vi "3.labtask4 (1).vi"() -> ()   [LabVIEW 2022 SP3]
uses:
  <vilib>/Utility/file.llb/Write Delimited Spreadsheet (DBL).vi
panel:
  out "Array":dbl[](array[numeric])
  in  "file path (dialog if empty)":path
  out "Waveform Chart":dynamicdata(graph)
  out "Total execution time (s)":u32
  out "Sampling period (ms)":dbl
  out "Total number of samples":dbl
  in  "Sampling rate (Hz)":dbl
  in  "Total duration (s)":dbl
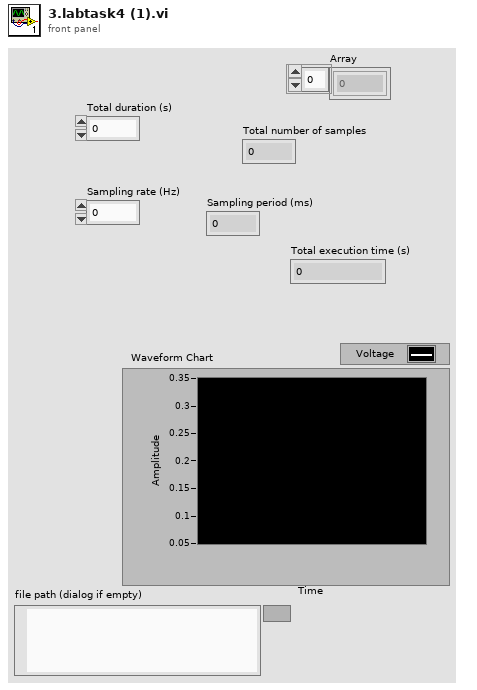
[diagram p1: front panel]
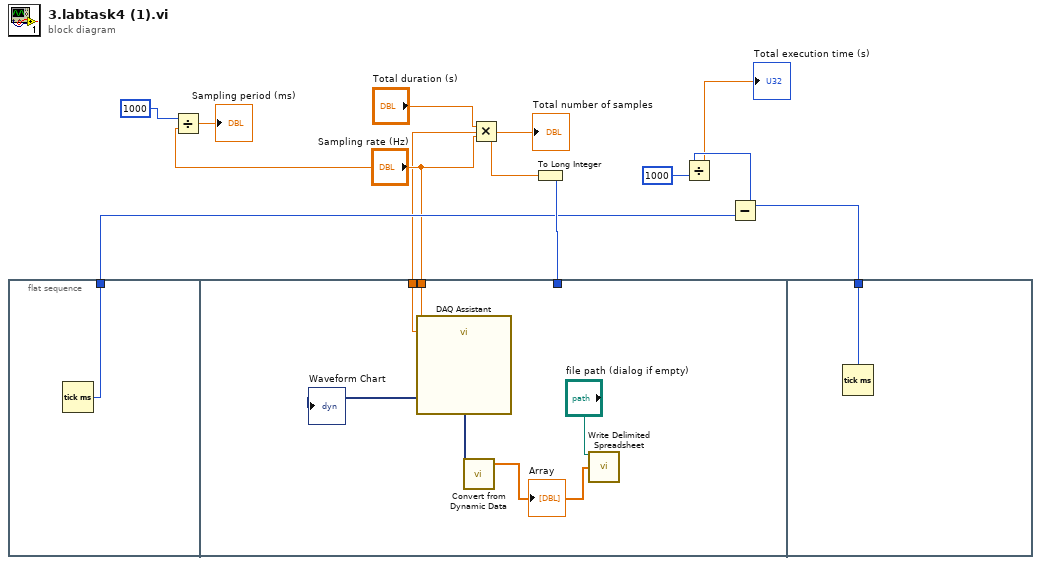
[diagram p0: block diagram]
diagram:
  n1 = flat-sequence {
    tunnel: [w12] -> w4
    tunnel: w9 -> [_]
    tunnel: "Sampling rate (Hz)" -> [w17]
    tunnel: w1 -> [w16]
    tunnel: [w18] -> w5
    frame #0 {
      n2 = Tick Count (ms)() -> (millisecond timer value=w12:u32)
    }
    frame #1 {
      n3 = call "DAQ Assistant"("rate"=w17, "number of samples"=w16) -> ("data"=w13:dynamicdata)  [unwired: 15 in, 2 out]
      "Waveform Chart" <- w13
      n4 = call "Convert from Dynamic Data"("Dynamic Data Type"=w13) -> ("Array"=w14:dbl[])  [unwired: 3 in]
      "Array" <- w14
      n5 = call-poly <vilib>:"Write Delimited Spreadsheet.vi"("file path (dialog if empty)"="file path (dialog if empty)", "1D data"=w14) -> ()  [unwired: 12 in, 2 out]
    }
    frame #2 {
      n6 = Tick Count (ms)() -> (millisecond timer value=w18:u32)
    }
  }
  n7 = Divide(x=1000, y="Sampling rate (Hz)") -> (x/y=→"Sampling period (ms)":dbl)
  n8 = Multiply(x="Total duration (s)", y="Sampling rate (Hz)") -> (x*y=w1:dbl)
  "Total number of samples" <- w1
  n9 = To Long Integer(number=w1) -> (32bit integer=w9:i32)
  n10 = Subtract(x=w5, y=w4) -> (x-y=w8:u32)
  n11 = Divide(x=w8, y=u32 1000) -> (x/y=→"Total execution time (s)":dbl)
